vi "Cleanup.vi"(8 "error in (no error)":errorcluster, 11 "Node in":refnum<class "bt_Parallel_Threaded.lvclass">) -> (0 "error out":errorcluster, 3 "Node out":refnum<class "bt_Parallel_Threaded.lvclass">)   [LabVIEW 2021, in "BT.lvlib" / "bt_Parallel_Threaded.lvclass"]
uses:
  bt_Parallel_Threaded.lvclass
  bt_Parallel_Threaded.lvclass/bt_Parallel_Threaded.ctl
  System/bt_System.lvclass
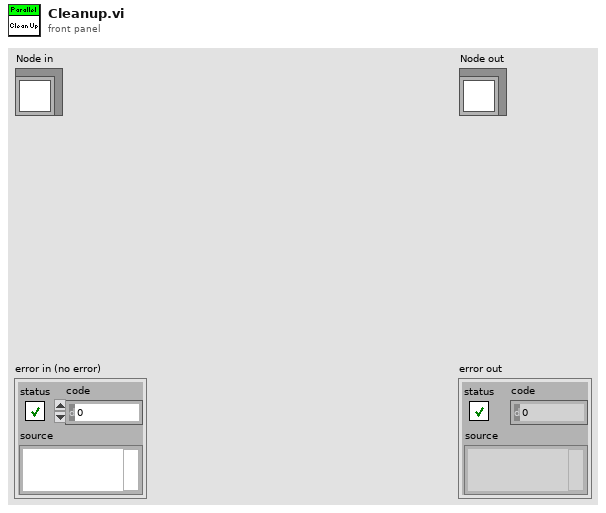
[diagram p1: front panel]
types:
  T1 = typedef "Rendezvous RefNum" = refnum<k1>
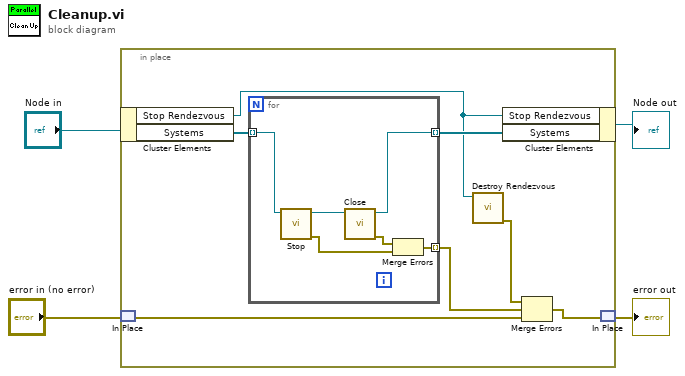
[diagram p0: block diagram]
diagram:
  n1 = in-place {
    n2 = in-place-cluster #1("Node in") -> ("Stop Rendezvous"=w6:T1, "Systems"=w11:refnum<class "bt_System.lvclass">[])
    n3 = in-place-match #2("error in (no error)") -> (w8:errorcluster)
    n4 = for {
      tunnel: w11 -> [w17] mode=indexing
      tunnel: [w15] -> w10 mode=indexing
      tunnel: [w12] -> w9 mode=indexing
      n5 = call "Stop.vi"("bt_System in"=w17) -> ("error out"=w13:errorcluster, "bt_System out"=w16:refnum<class "bt_System.lvclass">)  [unwired: 9 in]
      n6 = call-dynamic "Close.vi"("bt_System in"=w16) -> ("error out"=w14:errorcluster, "bt_System out"=w15:refnum<class "bt_System.lvclass">)  [unwired: 9 in]
      n7 = Merge Errors(w14, w13) -> (w12:errorcluster)
    }
    n8 = call <vilib>:"Destroy Rendezvous.vi"("rendezvous"=w6) -> ("error out"=w5:errorcluster)  [unwired: 5 in, 1 out]
    n9 = in-place-cluster #1("Stop Rendezvous"=w6, "Systems"=w10) -> (→"Node out":refnum<class "bt_Parallel_Threaded.lvclass">)
    n10 = Merge Errors(w5, w9, w8) -> (w7:errorcluster)
    n11 = in-place-match #2(w7) -> (→"error out":errorcluster)
  }
